vi "GUI_active_MotorForce.vi"(0 "lang":string, 3 "Total trial":u16=80 min=1) -> (8 "stop 2":bool)   [LabVIEW 2012]
uses:
  subVIs/Global_var.vi
  <vilib>/Analysis/1siggen.llb/Riffle Array (I32).vi
  <vilib>/Utility/file.llb/Write To Spreadsheet File (DBL).vi
  <userlib>/dhd_sdk7/dhd_sdk7.lvlib
  <vilib>/Analysis/NI_AALBase.lvlib
panel:
  in  "pause":bool
  out "Message":string="    Good. Don't give up!"
  out "Correct?":bool
  out "Trial_index":u16
  out "Trajectory":path
  out "Current seq":u8
  out "Target":dbl[](array[numeric])
  out "flag":bool
  out "Fz":dbl
  out "error out":errorcluster
  in  "Start?":bool
  out "Fx":dbl
  out "Fy":dbl
  out "Trial #":u16
  in  "stop":bool
  out "Canvas":picture
  # "Delta robot kinetics information"
  # "o"
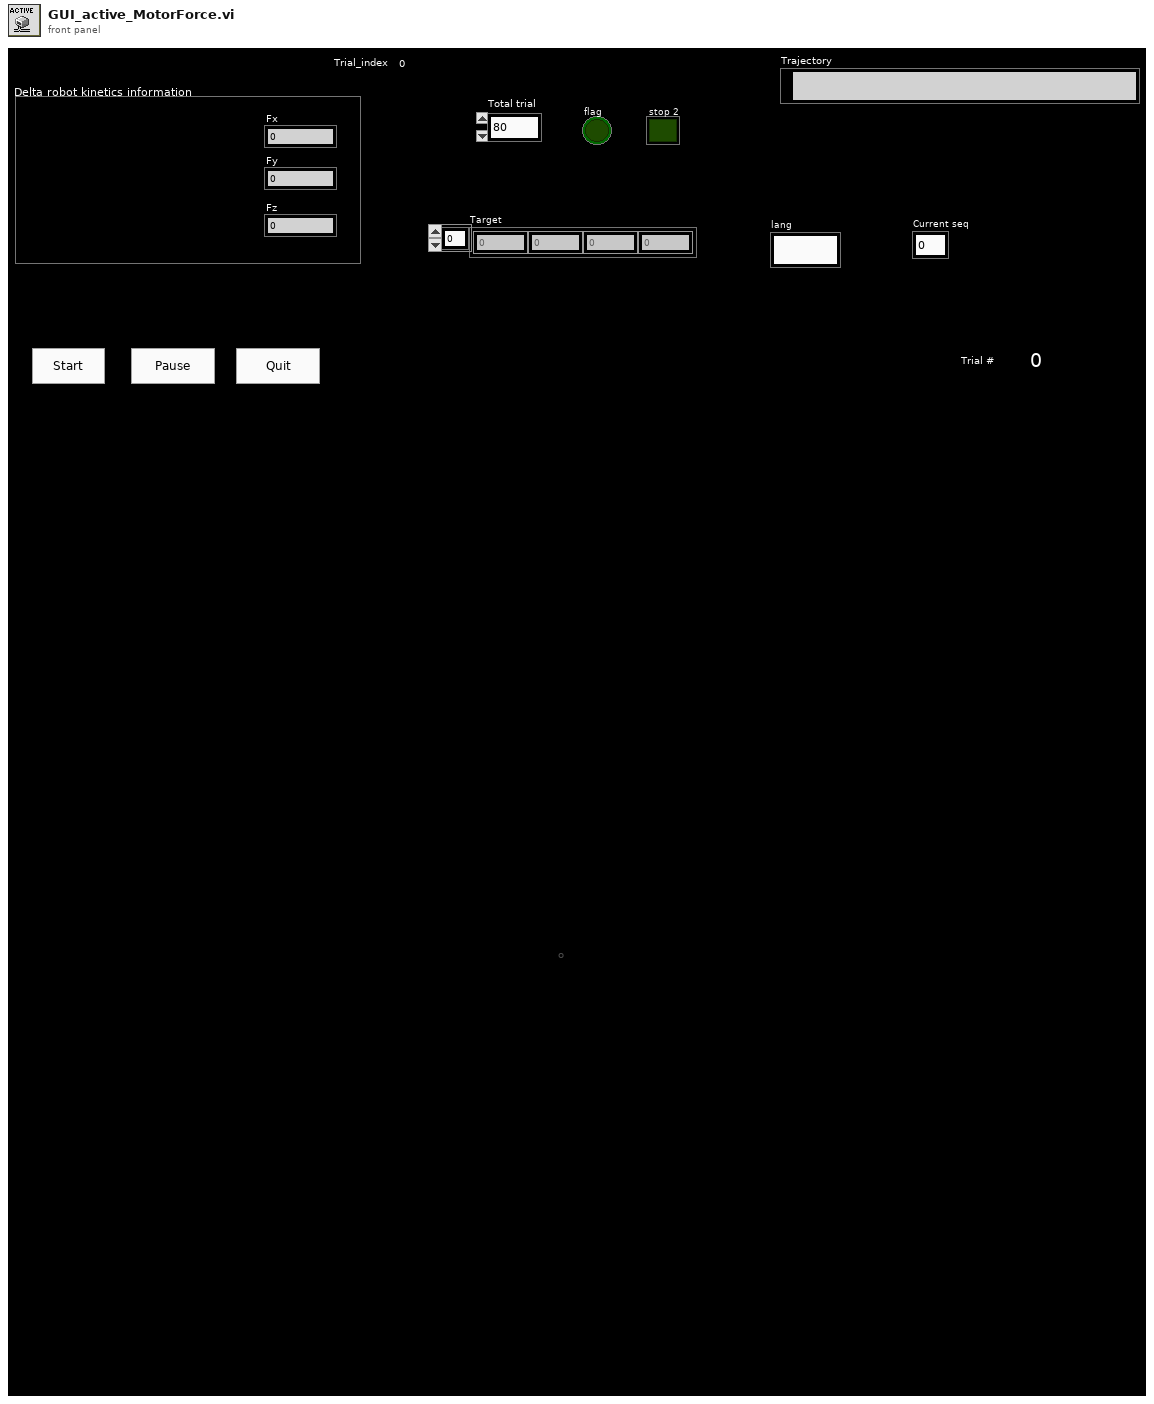
[diagram p1: front panel]
types:
  T1 = typedef "Sound Output Task ID.ctl" = u32
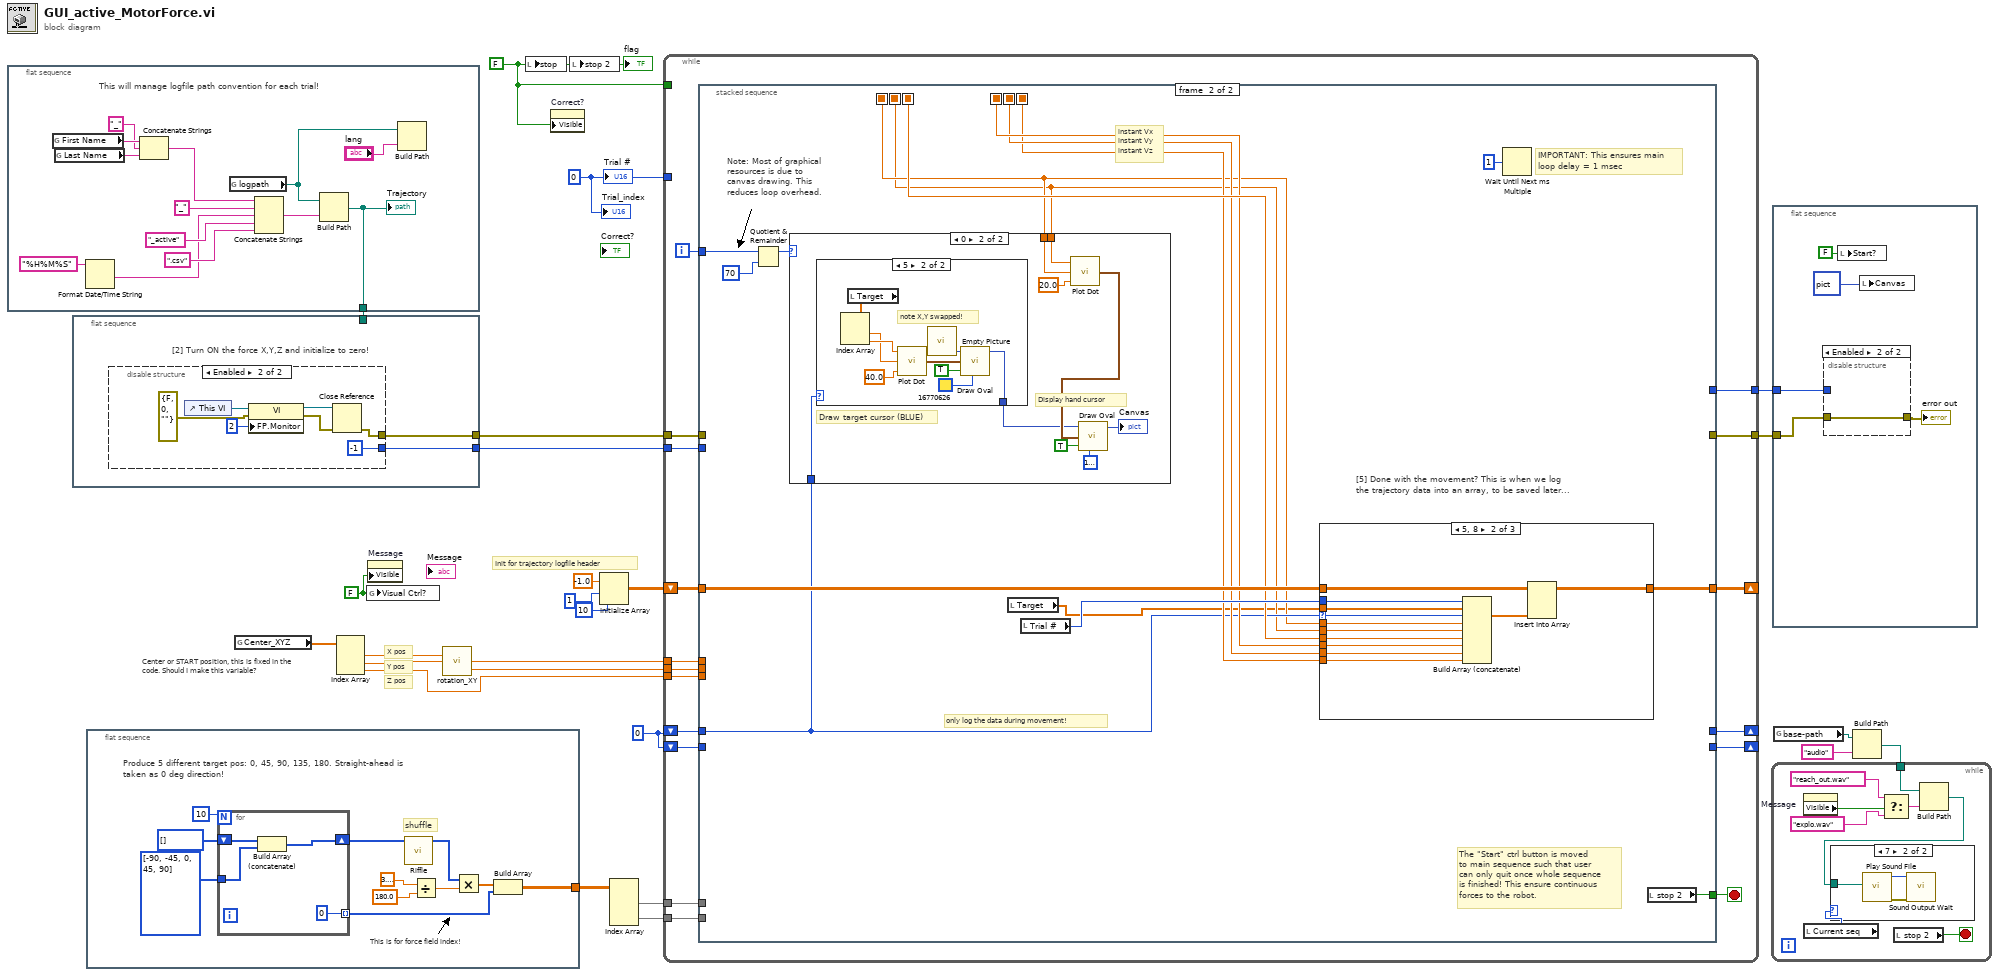
[diagram p0: block diagram]
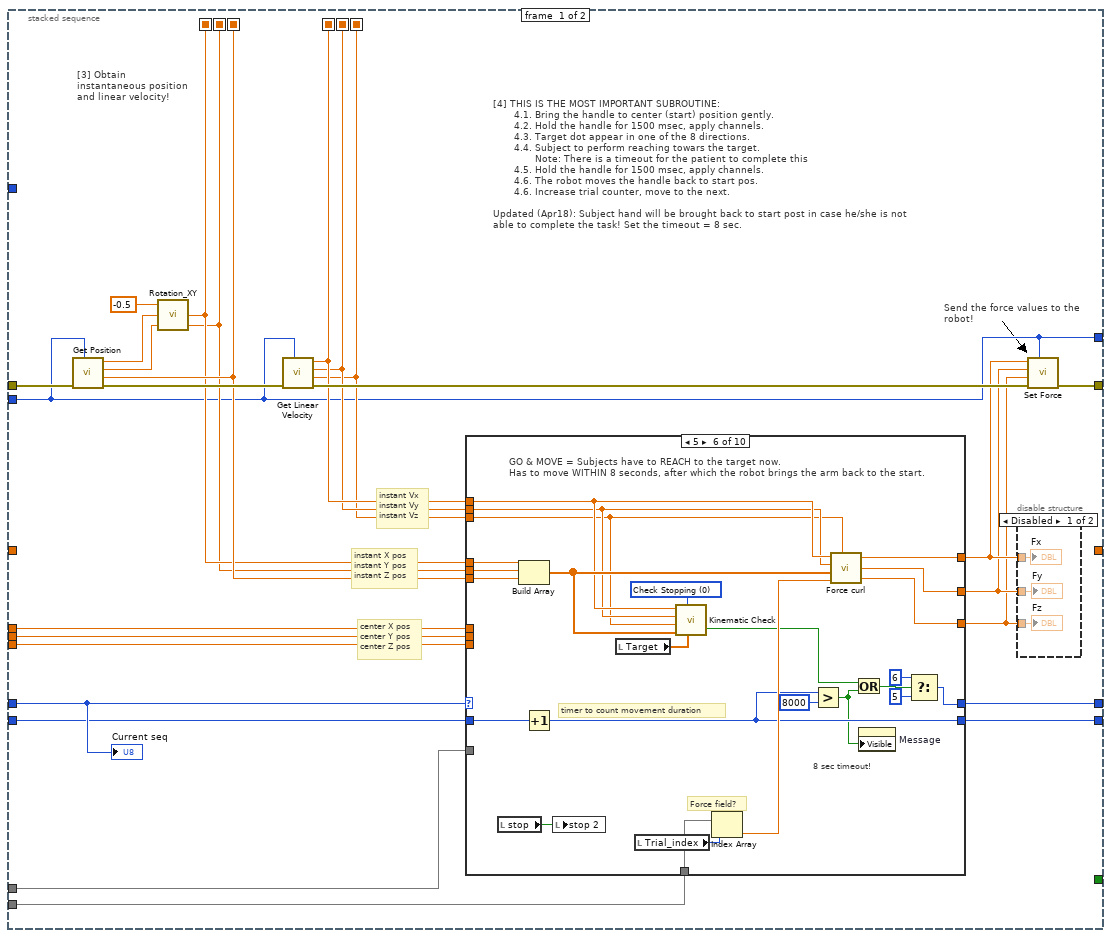
[diagram p3: hidden frame]
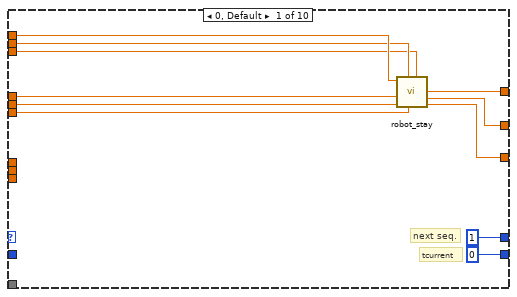
[diagram p5: hidden frame]
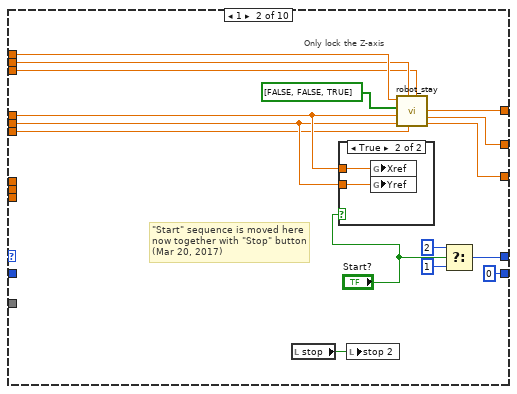
[diagram p6: hidden frame]
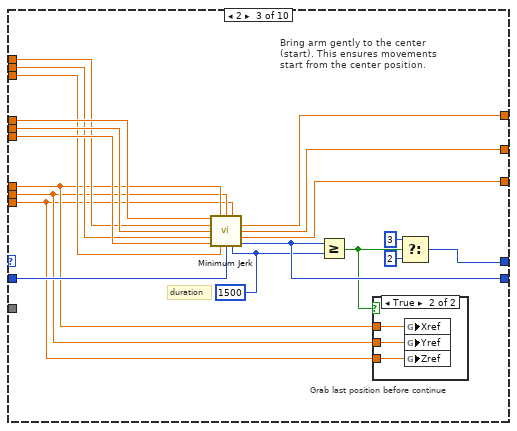
[diagram p8: hidden frame]
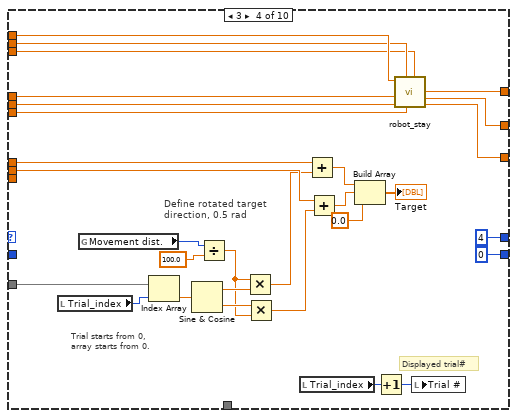
[diagram p10: hidden frame]
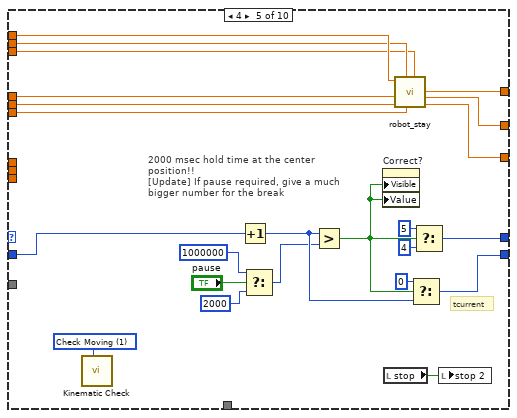
[diagram p11: hidden frame]
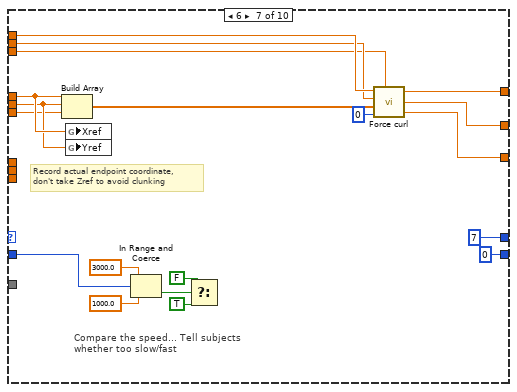
[diagram p12: hidden frame]
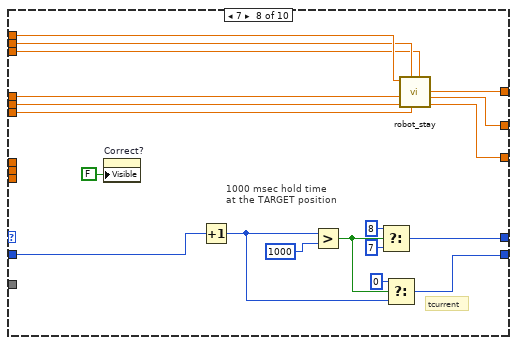
[diagram p13: hidden frame]
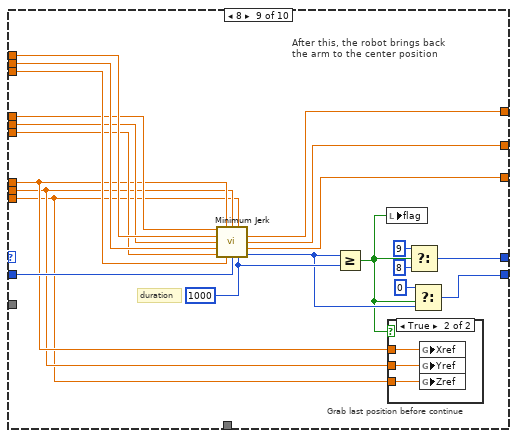
[diagram p14: hidden frame]
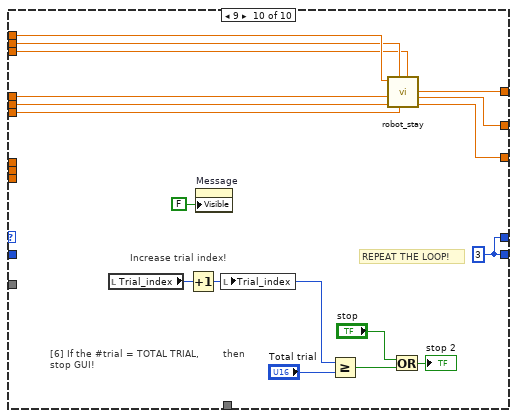
[diagram p16: hidden frame]
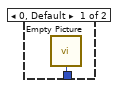
[diagram p18: hidden frame]
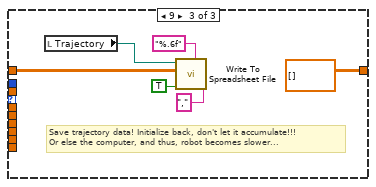
[diagram p20: hidden frame]
diagram:
  w4 = FALSE ("Visual Ctrl?")
  w15 = u16 0 ("y")
  w5 = FALSE ("stop")
  w22 = u16 0 ("ID")
  # "Z pos"
  # "Y pos"
  # "X pos"
  # "Center or START position, this is fixed in the code. Should I make this variable?"
  # "Init for trajectory logfile header"
  n1 = flat-sequence {
    tunnel: [w32] -> w20
    frame #0 {
      # "This will manage logfile path convention for each trial!"
      n2 = global read "Global_var.vi" "First Name"() -> (w30:string)
      n3 = global read "Global_var.vi" "Last Name"() -> (w28:string)
      n4 = Format Date/Time String(time format string (%c)="%H%M%S") -> (date/time string=w34:string)  [unwired: 2 in]
      n5 = Concatenate Strings(w30, "_" ("string"), w28) -> (w27:string)
      n6 = global read "Global_var.vi" "logpath"() -> (w26:path)
      n7 = Concatenate Strings(w27, "_" ("string"), w34, "_active" ("string"), ".csv" ("string")) -> (w38:string)
      n8 = Build Path(base path=w26, name or relative path=w38) -> (appended path=w32:path)
      "Trajectory" <- w32
      n9 = Build Path(base path=w26, name or relative path="lang") -> ()  [unwired: 1 out]
    }
  }
  n10 = flat-sequence {
    tunnel: [w40] -> w24
    tunnel: [w39] -> w23
    tunnel: w20 -> [_]
    frame #0 {
      # "[2] Turn ON the force X,Y,Z and initialize to zero!"
      n11 = disable-structure shown="Enabled" {
        disable-tunnel: [w42 w47] -> w40
        disable-tunnel: [w41 i8 -1 ("ID")] -> w39
        frame Disabled {
          w41 = i8 -1 ("ID")
          n12 = call <userlib>:"Open.vi"("error in (no error)"=errorcluster {"status"=FALSE, "code"=0, "source"=""} ("error out")) -> ("error out"=w43:errorcluster)  [unwired: 9 in, 1 out]
          n13 = call <userlib>:"Enable Force.vi"("error in (no error)"=w43, "ID"=w41, "val"=u8 1) -> ("error out"=w42:errorcluster)  [unwired: 7 in, 1 out]
        }
        frame Enabled {
          n14 = control-ref of="This VI"() -> (w48:refnum<vi>)
          n15 = property class="VI"(reference=w48, error in=errorcluster {"status"=FALSE, "code"=0, "source"=""} ("error out"), "FP.Monitor"=u16 2 ("Front Panel Window:Monitor")) -> (reference out=w51:refnum<vi>, error out=w50:errorcluster)
          n16 = Close Reference(reference=w51, error in (no error)=w50) -> (error out=w47:errorcluster)
        }
      }
    }
  }
  n17 = flat-sequence {
    tunnel: [w54] -> w8
    frame #0 {
      # "This is for force field index!"
      # "Produce 5 different target pos: 0, 45, 90, 135, 180. Straight-ahead is taken as 0 deg direction!"
      # "shuffle"
      n18 = for {
        N: 10 -> [_]
        shift-right: [w67] -> w56
        shift-left: i32[] [] -> [w65]
        tunnel: i32[] [-90, -45, 0, 45, 90] -> [w66]
        tunnel: [0] -> w53 mode=indexing
        n19 = Build Array (concatenate)(w65, w66) -> (w67:i32[])
      }
      n20 = call-poly <vilib>:"Riffle.vi"("X"=w56) -> ("Riffled {X}"=w63:i32[])  [unwired: 8 in, 2 out]
      n21 = Divide(x=3.141592653589793, y=180.0) -> (x/y=w61:dbl)
      n22 = Multiply(x=w63, y=w61) -> (x*y=w55:dbl[])
      n23 = Build Array(w55, w53) -> (w54:dbl[][])
    }
  }
  n24 = global read "Global_var.vi" "Center_XYZ"() -> (w12:dbl[])
  n25 = Index Array(array=w12) -> (element #1=w14:dbl, element #2=w13:dbl, element #3=w11:dbl)  [unwired: 3 in]
  n26 = global write "Global_var.vi" "Visual Ctrl?"(w4) -> ()
  n27 = property on="Message" class="Str"("Visible"=w4) -> ()  [unwired: 2 in, 2 out]
  n28 = call "rotation_XY.vi"("x_pos"=w13, "angle"=w14) -> ("rot_y"=w10:dbl, "rot_x"=w9:dbl)  [unwired: 2 in]
  n29 = local write "stop"(w5) -> ()
  n30 = property on="Correct?" class="Bool (strict)"("Visible"=w5) -> ()  [unwired: 2 in, 2 out]
  n31 = local write "stop 2"(w5) -> ()
  n32 = Initialize Array(-1.0 ("vz out"), 1 ("dimension size"), 10 ("dimension size")) -> (w19:dbl[][])
  n33 = Index Array(array=w8) -> (element #1=w7:dbl[], element #2=w6:dbl[])  [unwired: 4 in]
  n34 = while {
    tunnel: w23 -> [w83]
    shift-right: [w84] -> _
    shift-left: w22 -> [w79]
    shift-right: [w81] -> _
    shift-left: w19 -> [w80]
    tunnel: [w77] -> w25
    tunnel: w15 -> [_]
    tunnel: w24 -> [w76]
    shift-right: [w74] -> _
    shift-left: w22 -> [w75]
    tunnel: w5 -> [_]
    tunnel: [w73] -> w21
    tunnel: w9 -> [w72]
    tunnel: w10 -> [w71]
    tunnel: w11 -> [w70]
    tunnel: w7 -> [w69]
    tunnel: w6 -> [w68]
    i -> [w78]
    stop <- w82 stop-if-true
    n35 = stacked-sequence {
      seq-local: [w99 _] -> [_ w330]
      seq-local: [w96 _] -> [_ w327]
      seq-local: [w98 _] -> [_ w329]
      seq-local: [w97 _] -> [_ w328]
      seq-local: [w88 _] -> [_ w323]
      seq-local: [w89 _] -> [_ w324]
      tunnel: [w109 _] -> w84
      tunnel: w83 -> [w85 _]
      tunnel: [_ w322] -> w82
      tunnel: [_ w333] -> w81
      tunnel: w80 -> [_ w332]
      tunnel: w79 -> [w110 w325]
      tunnel: w78 -> [_ w335]
      tunnel: [w85 _] -> w77
      tunnel: w76 -> [w104 _]
      tunnel: w75 -> [w108 _]
      tunnel: [w107 _] -> w74
      tunnel: [w106 _] -> w73
      tunnel: w72 -> [w95 _]
      tunnel: w71 -> [w94 _]
      tunnel: w70 -> [w93 _]
      tunnel: w69 -> [w87 _]
      tunnel: w68 -> [w86 _]
      frame #0 {
        # "[4] THIS IS THE MOST IMPORTANT SUBROUTINE:\n       4.1. Bring the handle to center (start) position gently.\n       4.2. Hold the handle for 1500 msec, apply channels.\n       4.3. Target dot appear in one of the 8 directions.\n       4.4. Subject to perform reaching towars the target.\n              Note: There is a timeout for the patient to complete this\n       4.5. Hold the handle for 1500 msec, apply channels.\n       4.6. The robot moves the handle back to start pos.\n       4.6. Increase trial counter, move to the next.\n\nUpdated (Apr18): Subject hand will be brought back to start post in case he/she is not able to complete the task! Set the timeout = 8 sec."
        # "center X pos\ncenter Y pos\ncenter Z pos"
        # "[3] Obtain instantaneous position and linear velocity!"
        # "Send the force values to the robot!"
        # "instant Vx\ninstant Vy\ninstant Vz"
        # "instant X pos\ninstant Y pos\ninstant Z pos"
        n36 = call <userlib>:"Get Position.vi"("ID"=w85, "error in (no error)"=w104) -> ("error out"=w105:errorcluster, "pz out"=w99:dbl, "py out"=w90:dbl, "px out"=w91:dbl)  [unwired: 5 in, 1 out]
        n37 = call "Rotation_XY.vi"("y_pos"=w90, "x_pos"=w91, "angle"=-0.5) -> ("rot_y"=w88:dbl, "rot_x"=w89:dbl)  [unwired: 1 in]
        n38 = call <userlib>:"Get Linear Velocity.vi"("ID"=w85, "error in (no error)"=w105) -> ("error out"=w103:errorcluster, "vz out"=w96:dbl, "vy out"=w97:dbl, "vx out"=w98:dbl)  [unwired: 5 in, 1 out]
        n39 = case shown="5" w110 {
          tunnel: [u8 1 ("ID") w131 w159 u8 4 ("ID") w214 w234 u32 7 ("ID") w276 w287 w320] -> w109
          tunnel: [w116 w136 w155 w176 w203 w237 w260 w264 w291 w312] -> w102
          tunnel: [w115 w135 w156 w175 w202 w236 w259 w263 w290 w311] -> w101
          tunnel: w108 -> [_ _ w153 _ w211 w222 w244 w272 w288 _]
          tunnel: [u16 0 ("tcurrent") u32 0 ("ID") w158 u32 0 ("ID") w212 w218 u32 0 ("ID") w274 w284 w320] -> w107
          tunnel: [w114 w134 w157 w174 w201 w235 w258 w262 w289 w310] -> w100
          tunnel: w89 -> [w119 w128 w152 w179 w206 w232 w256 w267 w294 w315]
          tunnel: w88 -> [w118 w127 w151 w178 w205 w231 w255 w266 w293 w314]
          tunnel: w99 -> [w117 w126 w150 w177 w204 w230 w254 w265 w292 w313]
          tunnel: w98 -> [w122 w139 w149 w182 w209 w226 w252 w270 w297 w318]
          tunnel: w97 -> [w121 w138 w148 w181 w208 w225 w251 w269 w296 w317]
          tunnel: w96 -> [w120 w137 w147 w180 w207 w224 w250 w268 w295 w316]
          tunnel: w95 -> [_ _ w145 w169 _ _ _ _ w282 _]
          tunnel: w94 -> [_ _ w144 w168 _ _ _ _ w281 _]
          tunnel: w93 -> [_ _ w143 _ _ _ _ _ w280 _]
          tunnel: w87 -> [_ _ _ w167 _ _ _ _ _ _]
          tunnel: w86 -> [_ _ _ _ _ w238 _ _ _ _]
          frame 0, Default {
            # "next seq."
            # "tcurrent"
            n40 = call "robot_stay.vi"("Vz"=w120, "Z"=w117, "Vy"=w121, "Y"=w118, "X"=w119, "Vx"=w122) -> ("Fz"=w114:dbl, "Fy"=w115:dbl, "Fx"=w116:dbl)  [unwired: 3 in]
          }
          frame 1 {
            # "Only lock the Z-axis"
            # "\"Start\" sequence is moved here \nnow together with \"Stop\" button\n(Mar 20, 2017)"
            n41 = local read "stop"() -> (w130:bool)
            n42 = case shown="True" "Start?" {
              tunnel: w128 -> [_ w142]
              tunnel: w127 -> [_ w141]
              frame False {
              }
              frame True {
                n43 = global write "Global_var.vi" "Xref"(w142) -> ()
                n44 = global write "Global_var.vi" "Yref"(w141) -> ()
              }
            }
            n45 = local write "stop 2"(w130) -> ()
            n46 = call "robot_stay.vi"("Vz"=w137, "Z"=w126, "Vy"=w138, "Y"=w127, "X"=w128, "Active?"=bool[] [FALSE, FALSE, TRUE], "Vx"=w139) -> ("Fz"=w134:dbl, "Fy"=w135:dbl, "Fx"=w136:dbl)  [unwired: 2 in]
            n47 = Select(t=u8 2, s="Start?", f=u8 1) -> (s? t:f=w131:u8)
          }
          frame 2 {
            w154 = u16 1500 ("duration")
            # "Grab last position before continue"
            # "Bring arm gently to the center\n(start). This ensures movements\nstart from the center position."
            # "duration"
            n48 = call "Minimum Jerk.vi"("X"=w152, "Xfinal"=w145, "Yfinal"=w144, "Zfinal"=w143, "Vx"=w149, "Y"=w151, "Vy"=w148, "Z"=w150, "Vz"=w147, "current_n"=w153, "duration"=w154) -> ("Fx"=w155:dbl, "Fy"=w156:dbl, "Fz"=w157:dbl, "n out"=w158:u16)  [unwired: 1 out]
            n49 = Greater Or Equal?(x=w158, y=w154) -> (x >= y?=w146:bool)
            n50 = case shown="True" w146 {
              tunnel: w145 -> [_ w164]
              tunnel: w144 -> [_ w163]
              tunnel: w143 -> [_ w162]
              frame False {
              }
              frame True {
                n51 = global write "Global_var.vi" "Xref"(w164) -> ()
                n52 = global write "Global_var.vi" "Yref"(w163) -> ()
                n53 = global write "Global_var.vi" "Zref"(w162) -> ()
              }
            }
            n54 = Select(t=u8 3 ("ID"), s=w146, f=u8 2) -> (s? t:f=w159:u8)
          }
          frame 3 {
            # "Displayed trial#"
            # "Trial starts from 0,\narray starts from 0."
            # "Define rotated target direction, 0.5 rad"
            n55 = local read "Trial_index"() -> (w189:u16)
            n56 = global read "Global_var.vi" "Movement dist."() -> (w186:u8)
            n57 = Index Array(array=w167, index=w189) -> (element=w190:dbl)
            n58 = Sine & Cosine(0:w190) -> (1:w191:dbl, 2:w192:dbl)
            n59 = Divide(x=w186, y=100.0) -> (x/y=w184:dbl)
            n60 = Multiply(x=w184, y=w191) -> (x*y=w166:dbl)
            n61 = Multiply(x=w192, y=w184) -> (x*y=w165:dbl)
            n62 = local read "Trial_index"() -> (w187:u16)
            n63 = Add(x=w169, y=w166) -> (x+y=w172:dbl)
            n64 = Add(x=w168, y=w165) -> (x+y=w171:dbl)
            n65 = Build Array(w172, w171, 0.0 ("element")) -> (→"Target":dbl[])
            n66 = Increment(x=w187) -> (x+1=w188:u16)
            n67 = call "robot_stay.vi"("Vz"=w180, "Z"=w177, "Vy"=w181, "Y"=w178, "X"=w179, "Vx"=w182) -> ("Fz"=w174:dbl, "Fy"=w175:dbl, "Fx"=w176:dbl)  [unwired: 3 in]
            n68 = local write "Trial #"(w188) -> ()
          }
          frame 4 {
            w199 = u16 1 items=["Check Stopping", "Check Moving", "Reached Dest."] ("Selection")
            # "2000 msec hold time at the center position!!\n[Update] If pause required, give a much bigger number for the break"
            # "tcurrent"
            n69 = call "Kinematic Check.vi"("Selection"=w199) -> ()  [unwired: 5 in, 2 out]
            n70 = Increment(x=w211) -> (x+1=w210:u32)
            n71 = Select(t=u32 1000000 ("y"), s="pause", f=u32 2000 ("y")) -> (s? t:f=w195:u32)
            n72 = Greater?(x=w210, y=w195) -> (0:w200:bool)
            n73 = property on="Correct?" class="Bool (strict)"("Visible"=w200, "Value"=w200) -> ()  [unwired: 2 in, 2 out]
            n74 = local read "stop"() -> (w194:bool)
            n75 = call "robot_stay.vi"("Vz"=w207, "Z"=w204, "Vy"=w208, "Y"=w205, "X"=w206, "Vx"=w209) -> ("Fz"=w201:dbl, "Fy"=w202:dbl, "Fx"=w203:dbl)  [unwired: 3 in]
            n76 = Select(t=u8 0 ("ID"), s=w200, f=w210) -> (s? t:f=w212:u32)
            n77 = Select(t=u8 5 ("ID"), s=w200, f=u8 4) -> (s? t:f=w214:u8)
            n78 = local write "stop 2"(w194) -> ()
          }
          frame 5 {
            w227 = u16 0 items=["Check Stopping", "Check Moving", "Reached Dest."] ("Selection")
            # "8 sec timeout!"
            # "timer to count movement duration"
            # "Force field?"
            # "GO & MOVE = Subjects have to REACH to the target now. \nHas to move WITHIN 8 seconds, after which the robot brings the arm back to the start."
            n79 = local read "stop"() -> (w223:bool)
            n80 = Build Array(w232, w231, w230) -> (w228:dbl[])
            n81 = Increment(x=w222) -> (x+1=w218:u32)
            n82 = local write "stop 2"(w223) -> ()
            n83 = local read "Target"() -> (w229:dbl[])
            n84 = local read "Trial_index"() -> (w233:u16)
            n85 = call "Kinematic Check.vi"("Ref_pos"=w229, "Selection"=w227, "Inst_pos"=w228, "Vz"=w224, "Vy"=w225, "Vx"=w226) -> ("True?"=w219:bool)  [unwired: 1 out]
            n86 = Index Array(array=w238, index=w233) -> (element=w241:dbl)
            n87 = Greater?(x=w218, y=u32 8000) -> (0:w217:bool)
            n88 = call "Force curl.vi"("Vx"=w226, "Vz"=w224, "Vy"=w225, "Instant_pos"=w228, "Type"=w241) -> ("Fx"=w237:dbl, "Fy"=w236:dbl, "Fz"=w235:dbl)  [unwired: 1 in]
            n89 = Or(x=w219, y=w217) -> (x .or. y?=w220:bool)
            n90 = property on="Message" class="Str"("Visible"=w217) -> ()  [unwired: 2 in, 2 out]
            n91 = Select(t=u8 6 ("ID"), s=w220, f=u8 5) -> (s? t:f=w234:u8)
          }
          frame 6 {
            # "Record actual endpoint coordinate,\ndon't take Zref to avoid clunking"
            # "Compare the speed... Tell subjects \nwhether too slow/fast"
            n92 = Build Array(w256, w255, w254) -> (w253:dbl[])
            n93 = global write "Global_var.vi" "Xref"(w256) -> ()
            n94 = global write "Global_var.vi" "Yref"(w255) -> ()
            n95 = In Range and Coerce(upper limit=3000.0, x=w244, lower limit=1000.0) -> (In Range?=w245:bool)  [unwired: 1 out]
            n96 = Select(t=FALSE ("Visual Ctrl?"), s=w245, f=TRUE ("Visual Ctrl?")) -> ()  [unwired: 1 out]
            n97 = call "Force curl.vi"("Vx"=w252, "Vz"=w250, "Vy"=w251, "Instant_pos"=w253, "Type"=u16 0) -> ("Fx"=w260:dbl, "Fy"=w259:dbl, "Fz"=w258:dbl)  [unwired: 1 in]
          }
          frame 7 {
            # "1000 msec hold time\nat the TARGET position"
            # "tcurrent"
            n98 = property on="Correct?" class="Bool (strict)"("Visible"=FALSE ("Correct?")) -> ()  [unwired: 2 in, 2 out]
            n99 = Increment(x=w272) -> (x+1=w271:u32)
            n100 = Greater?(x=w271, y=u32 1000) -> (0:w273:bool)
            n101 = Select(t=u8 8 ("ID"), s=w273, f=u8 7) -> (s? t:f=w276:u8)
            n102 = Select(t=u8 0 ("ID"), s=w273, f=w271) -> (s? t:f=w274:u32)
            n103 = call "robot_stay.vi"("Vz"=w268, "Z"=w265, "Vy"=w269, "Y"=w266, "X"=w267, "Vx"=w270) -> ("Fz"=w262:dbl, "Fy"=w263:dbl, "Fx"=w264:dbl)  [unwired: 3 in]
          }
          frame 8 {
            w298 = u16 1000 ("duration")
            # "Grab last position before continue"
            # "After this, the robot brings back\nthe arm to the center position"
            # "duration"
            n104 = call "Minimum Jerk.vi"("X"=w294, "Xfinal"=w282, "Yfinal"=w281, "Zfinal"=w280, "Vx"=w297, "Y"=w293, "Vy"=w296, "Z"=w292, "Vz"=w295, "current_n"=w288, "duration"=w298) -> ("Fx"=w291:dbl, "Fy"=w290:dbl, "Fz"=w289:dbl, "n out"=w285:u16)  [unwired: 1 out]
            n105 = Greater Or Equal?(x=w285, y=w298) -> (x >= y?=w283:bool)
            n106 = local write "flag"(w283) -> ()
            n107 = case shown="True" w283 {
              tunnel: w282 -> [_ w303]
              tunnel: w281 -> [_ w302]
              tunnel: w280 -> [_ w301]
              frame False {
              }
              frame True {
                n108 = global write "Global_var.vi" "Xref"(w303) -> ()
                n109 = global write "Global_var.vi" "Yref"(w302) -> ()
                n110 = global write "Global_var.vi" "Zref"(w301) -> ()
              }
            }
            n111 = Select(t=u8 9 ("ID"), s=w283, f=u8 8) -> (s? t:f=w287:u8)
            n112 = Select(t=u16 0, s=w283, f=w285) -> (s? t:f=w284:u16)
          }
          frame 9 {
            w320 = u8 3 ("ID")
            # "[6] If the #trial = TOTAL TRIAL,        then stop GUI!"
            # "Increase trial index!"
            # "REPEAT THE LOOP!"
            n113 = local read "Trial_index"() -> (w319:u16)
            n114 = Increment(x=w319) -> (x+1=w306:u16)
            n115 = property on="Message" class="Str"("Visible"=FALSE) -> ()  [unwired: 2 in, 2 out]
            n116 = local write "Trial_index"(w306) -> ()
            n117 = Greater Or Equal?(x=w306, y="Total trial") -> (x >= y?=w309:bool)
            n118 = call "robot_stay.vi"("Vz"=w316, "Z"=w313, "Vy"=w317, "Y"=w314, "X"=w315, "Vx"=w318) -> ("Fz"=w310:dbl, "Fy"=w311:dbl, "Fx"=w312:dbl)  [unwired: 3 in]
            n119 = Or(x="stop", y=w309) -> (x .or. y?=→"stop 2":bool)
          }
        }
        n120 = disable-structure shown="Disabled" {
          disable-tunnel: w102 -> [w113 _]
          disable-tunnel: w101 -> [w112 _]
          disable-tunnel: w100 -> [w111 _]
          frame Disabled {
            "Fy" <- w112
            "Fx" <- w113
            "Fz" <- w111
          }
          frame Enabled {
          }
        }
        n121 = call <userlib>:"Set Force.vi"("ID"=w85, "error in (no error)"=w103, "fz"=w100, "fy"=w101, "fx"=w102) -> ("error out"=w106:errorcluster)  [unwired: 5 in, 1 out]
        "Current seq" <- w110
      }
      frame #1 {
        # "The \"Start\" ctrl button is moved\nto main sequence such that user\ncan only quit once whole sequence\nis finished! This ensure continuous\nforces to the robot."
        # "instant Vx\ninstant Vy\ninstant Vz"
        # "Note: Most of graphical resources is due to canvas drawing. This\nreduces loop overhead."
        # "IMPORTANT: This ensures main \nloop delay = 1 msec"
        # "only log the data during movement!"
        # "[5] Done with the movement? This is when we log\nthe trajectory data into an array, to be saved later..."
        n122 = Quotient & Remainder(x=w335, y=70) -> (x-y*floor(x/y)=w326:i32)  [unwired: 1 out]
        n123 = case shown="0" w326 {
          tunnel: w324 -> [_ w337]
          tunnel: w323 -> [_ w338]
          tunnel: w325 -> [_ w339]
          frame 1, Default {
          }
          frame 0 {
            # "Draw target cursor (BLUE)"
            # "Display hand cursor"
            n124 = case shown="5" w339 {
              tunnel: [w346 w351] -> w341
              frame 0, Default {
                n125 = call "Empty Picture"() -> ("empty picture"=w346:picture)
              }
              frame 5 {
                # "note X,Y swapped!"
                n126 = local read "Target"() -> (w349:dbl[])
                n127 = Index Array(array=w349) -> (element #1=w347:dbl, element #2=w348:dbl)  [unwired: 2 in]
                n128 = call "Plot Dot.vi"("Diameter"=40.0 ("Size"), "Y"=w347, "X"=w348) -> ("Cluster"=w355:cluster{dbl, dbl, dbl, dbl})
                n129 = call "Empty Picture"() -> ("empty picture"=w352:picture)
                n130 = call <vilib>:"Draw Oval.vi"("picture"=w352, "rect"=w355, "fill?(F)"=TRUE, "color(black)"=u32 16770626) -> ("new picture"=w351:picture)  [unwired: 5 in]
              }
            }
            n131 = call "Plot Dot.vi"("Diameter"=20.0 ("Size"), "Y"=w337, "X"=w338) -> ("Cluster"=w344:cluster{dbl, dbl, dbl, dbl})
            n132 = call <vilib>:"Draw Oval.vi"("picture"=w341, "rect"=w344, "fill?(F)"=TRUE, "color(black)"=u32 16777226) -> ("new picture"=→"Canvas":picture)  [unwired: 5 in]
          }
        }
        n133 = local read "Target"() -> (w321:dbl[])
        n134 = local read "Trial #"() -> (w334:u16)
        n135 = case shown="5, 8" w325 {
          selector: w325 -> [_ w357 _]
          tunnel: [w356 w367 dbl[][] []] -> w333
          tunnel: w332 -> [w356 w366 w371]
          tunnel: w321 -> [_ w358 _]
          tunnel: w334 -> [_ w365 _]
          tunnel: w324 -> [_ w364 _]
          tunnel: w323 -> [_ w363 _]
          tunnel: w330 -> [_ w362 _]
          tunnel: w329 -> [_ w361 _]
          tunnel: w328 -> [_ w360 _]
          tunnel: w327 -> [_ w359 _]
          frame 0, Default {
          }
          frame 5, 8 {
            n136 = Build Array (concatenate)(w365, w358, w357, w364, w363, w362, w361, w360, w359) -> (w368:dbl[])
            n137 = Insert Into Array(array=w366, new element=w368) -> (w367:dbl[][])  [unwired: 2 in]
          }
          frame 9 {
            # "Save trajectory data! Initialize back, don't let it accumulate!!!\nOr else the computer, and thus, robot becomes slower..."
            n138 = local read "Trajectory"() -> (w374:path)
            n139 = call-poly <vilib>:"Write To Spreadsheet File.vi"("delimiter (\\t)"="," ("delimiter (\\t)"), "format (%.3f)"="%.6f", "append to file? (new file:F)"=TRUE, "2D data"=w371, "file path (dialog if empty)"=w374) -> ()  [unwired: 3 in, 1 out]
          }
        }
        n140 = Wait Until Next ms Multiple(millisecond multiple=u32 1) -> ()  [unwired: 1 out]
        n141 = local read "stop 2"() -> (w322:bool)
      }
    }
  }
  n142 = flat-sequence {
    tunnel: w25 -> [w379]
    tunnel: w21 -> [w376]
    frame #0 {
      n143 = disable-structure shown="Enabled" {
        disable-tunnel: w379 -> [w382 _]
        disable-tunnel: w376 -> [w381 w383]
        disable-tunnel: [w380 w383] -> w375
        frame Disabled {
          # "Close!"
          n144 = call <userlib>:"Close.vi"("error in (no error)"=w381, "ID"=w382) -> ("error out"=w380:errorcluster)  [unwired: 8 in, 1 out]
        }
        frame Enabled {
        }
      }
      "error out" <- w375
      n145 = local write "Start?"(FALSE ("start")) -> ()
      n146 = local write "Canvas"(picture data[5B] ("Canvas")) -> ()
    }
  }
  n147 = global read "Global_var.vi" "base-path"() -> (w2:path)
  n148 = Build Path(base path=w2, name or relative path="audio") -> (appended path=w1:path)
  n149 = while {
    tunnel: w1 -> [w388]
    stop <- w390 stop-if-true
    n150 = property on="Message" class="Str"() -> ("Visible"=w387:bool)  [unwired: 2 in, 2 out]
    n151 = local read "Current seq"() -> (w391:u8)
    n152 = Select(t="reach_out.wav" ("name or relative path"), s=w387, f="explo.wav" ("name or relative path")) -> (s? t:f=w389:string)
    n153 = local read "stop 2"() -> (w390:bool)
    n154 = Build Path(base path=w388, name or relative path=w389) -> (appended path=w384:path)
    n155 = case shown="7" w391 {
      tunnel: w384 -> [_ w392]
      frame 0, Default {
      }
      frame 7 {
        n156 = call <vilib>:"Play Sound File.vi"("path"=w392) -> ("error out"=w394:errorcluster, "task ID"=w393:T1)  [unwired: 9 in]
        n157 = call <vilib>:"Sound Output Wait.vi"("error in (no error)"=w394, "task ID"=w393) -> ()  [unwired: 8 in, 2 out]
      }
    }
  }
  "flag" <- w5
  "Trial #" <- w15
  "Trial_index" <- w15
